vi "Intro to Arrays.vi"() -> ()   [LabVIEW 2019]
panel:
  out "max index(es)":i32
  out "max value":dbl
  out "Element B":dbl
  in  "Index":i32
  out "Element A":dbl
  out "Array Size":i32
  out "Edited Array":dbl[](array[numeric])
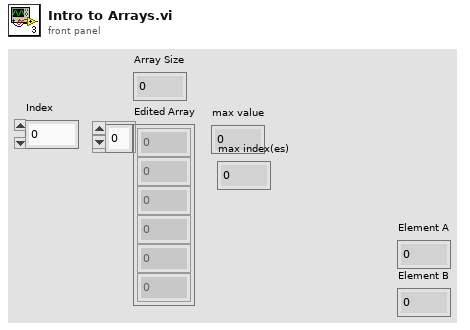
[diagram p1: front panel]
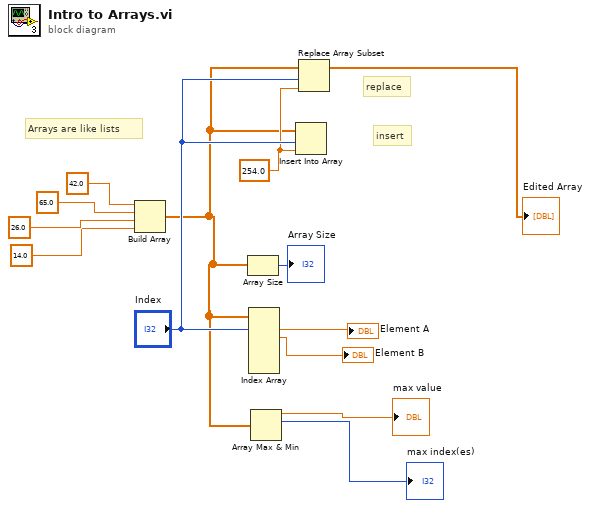
[diagram p0: block diagram]
diagram:
  w5 = 254.0 ("new element/subarray")
  # "insert"
  # "replace"
  # "Arrays are like lists"
  n1 = Build Array(42.0 ("element"), 65.0 ("element"), 26.0 ("element"), 14.0 ("element")) -> (w3:dbl[])
  n2 = Array Size(array=w3) -> (size(s)=→"Array Size":i32)
  n3 = Index Array(array=w3, index #1="Index") -> (element #1=→"Element A":dbl, element #2=→"Element B":dbl)  [unwired: 5 in, 4 out]
  n4 = Array Max & Min(array=w3) -> (max value=→"max value":dbl, max index (indices)=→"max index(es)":i32)  [unwired: 2 out]
  n5 = Insert Into Array(array=w3, index="Index", new element=w5) -> ()  [unwired: 1 out]
  n6 = Replace Array Subset(array=w3, new element=w5, index="Index") -> (→"Edited Array":dbl[])
